vi "NI OCR-Image Initialize_User Event.vi"(8 "error in":errorcluster, 11 "Buffer Data In":T1={"VI Refnum"=refnum, "Src Image"=refnum, "Dst Image"=refnum, "Ctl Refnum []"=[], "Ctl Label"=[], "User Event"=refnum, "Event Registration Refnum"=refnum, "Timeout"=0, "IMAQ OCR Session"=refnum, "Objects"=[], "ROI Descriptor"={"Global Rectangle"=[], "Contours"=[]}, "Settings"={"Objects"=0, "Threshold"=128, "Reject Border"=FALSE, "Fill Holes"=FALSE, "Min Object Size"=FALSE, "Min Size"=3, "Max Object Size"=FALSE, "Max Size"=100, "Show Search Area"=FALSE, "Show Center"=TRUE, "Show Bounding Box"=TRUE}} {"Settings"."Objects" items=["Bright Objects", "Dark Objects"]; "Settings"."Threshold" min=1 max=999999999 step=1; "Settings"."Max Size" min=1 max=999999999 step=1; "Settings"."Min Size" min=1 max=999999999 step=1; "ROI Descriptor"."Contours"."Type" items=["No Selection", "Point", "Line", "Rectangle", "Oval", "Polygon", "Freehand Region", "Annulus", "Unused2", "Unused3", "Broken Line", "Freehand Line", "Rotated Rectangle"]; "Objects"."Aspect Ratio" format="%.2f"; "Objects"."Orientation" format="%.2f"; "Objects"."Area" format="%.2f"; "Objects"."Object Center"."Y" format="%.2f"; "Objects"."Object Center"."X" format="%.2f"}) -> (0 "error out":errorcluster, 3 "Buffer Data Out":T1={"VI Refnum"=refnum, "Src Image"=refnum, "Dst Image"=refnum, "Ctl Refnum []"=[], "Ctl Label"=[], "User Event"=refnum, "Event Registration Refnum"=refnum, "Timeout"=0, "IMAQ OCR Session"=refnum, "Objects"=[], "ROI Descriptor"={"Global Rectangle"=[], "Contours"=[]}, "Settings"={"Objects"=0, "Threshold"=128, "Reject Border"=FALSE, "Fill Holes"=FALSE, "Min Object Size"=FALSE, "Min Size"=3, "Max Object Size"=FALSE, "Max Size"=100, "Show Search Area"=FALSE, "Show Center"=TRUE, "Show Bounding Box"=TRUE}} {"Settings"."Objects" items=["Bright Objects", "Dark Objects"]; "Settings"."Threshold" min=1 max=999999999 step=1; "Settings"."Max Size" min=1 max=999999999 step=1; "Settings"."Min Size" min=1 max=999999999 step=1; "ROI Descriptor"."Contours"."Type" items=["No Selection", "Point", "Line", "Rectangle", "Oval", "Polygon", "Freehand Region", "Annulus", "Unused2", "Unused3", "Broken Line", "Freehand Line", "Rotated Rectangle"]; "Objects"."Aspect Ratio" format="%.2f"; "Objects"."Orientation" format="%.2f"; "Objects"."Area" format="%.2f"; "Objects"."Object Center"."Y" format="%.2f"; "Objects"."Object Center"."X" format="%.2f"})   [LabVIEW 2016]
uses:
  Data Def/NI OCR-Buffer Data.ctl
  <vilib>/vision/Image Controls.llb/IMAQ Image.ctl
  Data Def/NI OCR-User Event Data.ctl
  <vilib>/vision/OCR.llb/IMAQ OCR Session.ctl
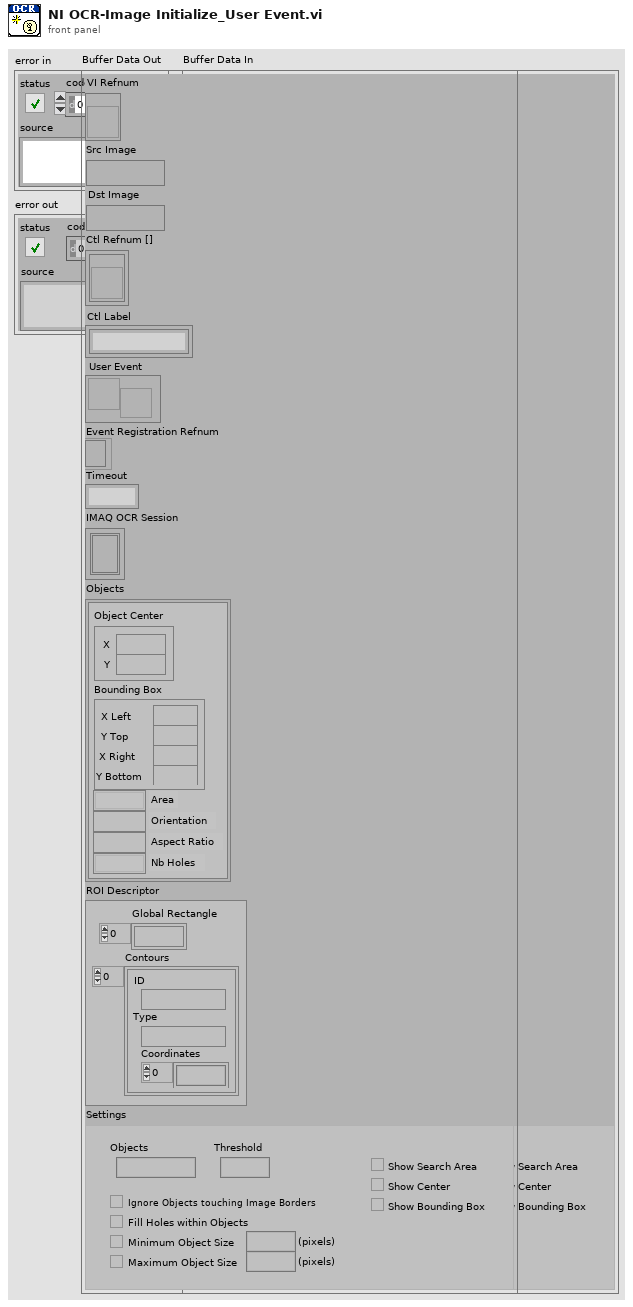
[diagram p1: front panel]
types:
  T1 = typedef "NI OCR-Buffer Data.ctl" = cluster{"VI Refnum":refnum<vi>, "Src Image":T2, "Dst Image":T2, "Ctl Refnum []":refnum<vi>[], "Ctl Label":string[], "User Event":refnum<user-event>, "Event Registration Refnum":refnum<event-registration>, "Timeout":i32, "IMAQ OCR Session":T3, "Objects":cluster{"Object Center":cluster{"X":sgl, "Y":sgl}, "Bounding Box":cluster{"X Left":i32, "Y Top":i32, "X Right":i32, "Y Bottom":i32}, "Area":sgl, "Orientation":sgl, "Aspect Ratio":sgl, "Nb Holes":i32}[], "ROI Descriptor":T4, "Settings":cluster{"Objects":u16, "Threshold":i32, "Reject Border":bool, "Fill Holes":bool, "Min Object Size":bool, "Min Size":i32, "Max Object Size":bool, "Max Size":i32, "Show Search Area":bool, "Show Center":bool, "Show Bounding Box":bool}}
  T2 = typedef "IMAQ Image.ctl" = refnum<image>
  T3 = typedef "IMAQ OCR Session.ctl" = refnum<k1>
  T4 = typedef "ROI Descriptor" = cluster{"Global Rectangle":i32[], "Contours":cluster{"ID":enum32{"External", "Internal"}, "Type":u32, "Coordinates":i32[]}[]}
  T5 = typedef "NI OCR-User Event Data.ctl" = cluster{"Command":string, "Data":variant}
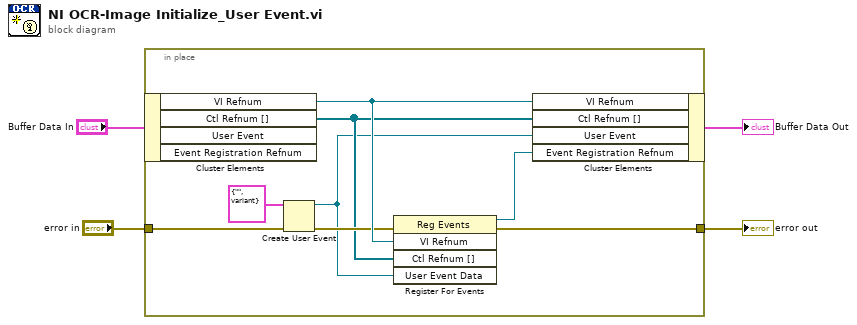
[diagram p0: block diagram]
diagram:
  n1 = in-place {
    in-place-border: "error in" -> [w9]
    in-place-border: [w6] -> w2
    n2 = in-place-cluster #1("Buffer Data In") -> ("VI Refnum"=w12:refnum<vi>, "Ctl Refnum []"=w10:refnum<vi>[])  [unwired: 2 out]
    n3 = Create User Event(user event datatype=T5 {"Command"="", "Data"=variant} ("User Event Data"), error in=w9) -> (user event=w7:refnum<user-event>, error out=w11:errorcluster)
    n4 = register-events(error in=w11, w12, w10, w7) -> (reference out=w5:refnum<event-registration>, error out=w6:errorcluster)  [unwired: 1 in]
    n5 = in-place-cluster #1("VI Refnum"=w12, "Ctl Refnum []"=w10, "User Event"=w7, "Event Registration Refnum"=w5) -> (→"Buffer Data Out":T1)
  }
  "error out" <- w2
